vi "thcd401_set_sp_value.vi"(5 "value":dbl, 7 "channel":u8=1 min=1 max=4 step=1, 8 "error in":errorcluster, 11 "conn_id_in":refnum<k5>) -> (0 "error out":errorcluster, 3 "conn_id_out":refnum<k5>, 4 "status":bool)   [LabVIEW 2019]
panel:
  out "query":string
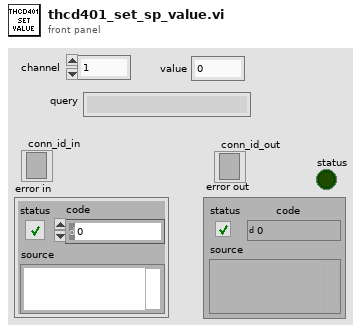
[diagram p1: front panel]
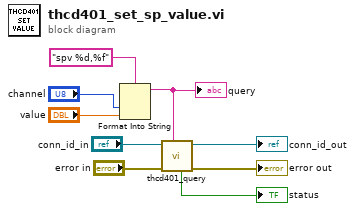
[diagram p0: block diagram]
diagram:
  n1 = Format Into String(format string="spv %d,%f", "channel", "value") -> (resulting string=w3:string)  [unwired: 2 in, 1 out]
  "query" <- w3
  n2 = call "thcd401_query.vi"("command"=w3, "error in"="error in", "conn_id_in"="conn_id_in") -> ("error out"=→"error out":errorcluster, "conn_id_out"=→"conn_id_out":refnum<k5>, "status"=→"status":bool)  [unwired: 5 in, 1 out]
